vi "Create Callback User Events.vi"(8 "error in":errorcluster, 11 "SourceGrid in":refnum<class "SourceGrid.lvclass">) -> (0 "error out":errorcluster, 3 "SourceGrid out":refnum<class "SourceGrid.lvclass">)   [LabVIEW 2024, in "SourceGrid.lvlib" / "SourceGrid.lvclass"]
uses:
  SourceGrid.lvclass
  MouseEventArgs/MouseEventArgs.lvclass
  SourceGrid.lvclass/SourceGrid.ctl
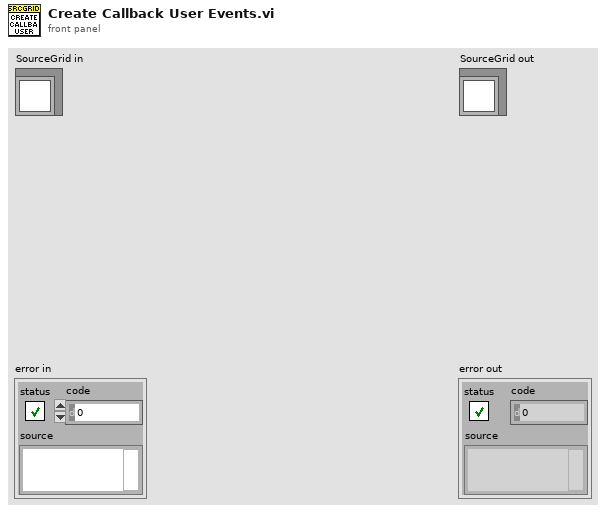
[diagram p1: front panel]
types:
  T1 = typedef "Rendezvous RefNum" = refnum<k1>
  T2 = cluster{"Context":refnum<class "MouseEventArgs.lvclass">, "rendezvous":T1}
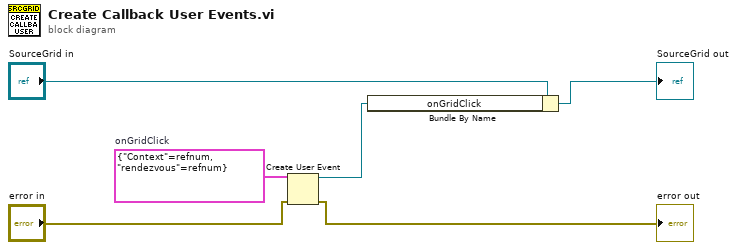
[diagram p0: block diagram]
diagram:
  w6 = T2 {"Context"=refnum, "rendezvous"=refnum}  # onGridClick
  n1 = Create User Event(user event datatype=w6, error in="error in") -> (user event=w1:refnum<user-event>, error out=→"error out":errorcluster)
  n2 = Bundle By Name(cluster="SourceGrid in", "onGridClick"=w1) -> (→"SourceGrid out":refnum<class "SourceGrid.lvclass">)
